vi "Example.vi"() -> ()   [LabVIEW 2020]
doc: "Modbus RTU for Invertek drives. Paul Nathan 21-JUN-2022."
uses:
  ctls/Drive address.ctl
  ctls/Modbus error cluster.ctl
  ctls/Exception codes.ctl
panel:
  out "No errors":bool
  out "Modbus error cluster":T1={"Checksum ok"=FALSE, "Modbus exception code"=1, "Response from correct drive"=FALSE, "Comms error"={"status"=FALSE, "code"=0, "source"=""}} {"Modbus exception code" items=["None"=0, "Invalid function request"=1, "Invalid Modbus register address"=2, "Invalid / unauthorised data value"=3, "Device failure"=4, "Request accepted, wait"=5, "Drive busy"=6, "Request rejected"=7, "Memory parity error"=8, "Gateway path unavailable"=10, "Device failed to respond"=11]}
  out "Motor power (kW)":dbl
  in  "Drive address":T3=1 items=["0", "1", "2", "3", "4", "5", "6", "7", "8", "9", "10", "11", "12", "13", "14", "15", "16", "17", "18", "19", "20", "21", "22", "23", "24", "25", "26", "27", "28", "29", "30", "31", "32", "33", "34", "35", "36", "37", "38", "39", "40", "41", "42", "43", "44", "45", "46", "47", "48", "49", "50", "51", "52", "53", "54", "55", "56", "57", "58", "59", "60", "61", "62", "63"]
  in  "COM port":refnum<visa-resource-name>
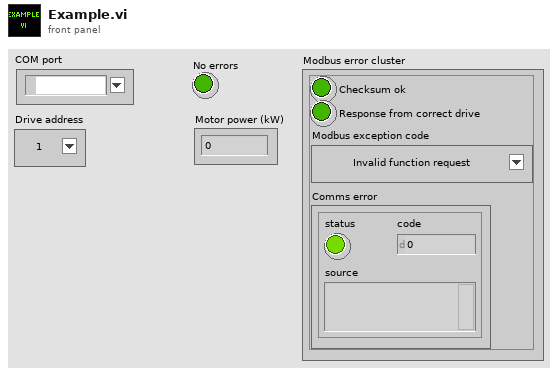
[diagram p1: front panel]
types:
  T1 = typedef "Modbus error cluster.ctl" = cluster{"Checksum ok":bool, "Modbus exception code":T2, "Response from correct drive":bool, "Comms error":errorcluster}
  T2 = typedef "Exception codes.ctl" = u8
  T3 = typedef "Drive address.ctl" = u8
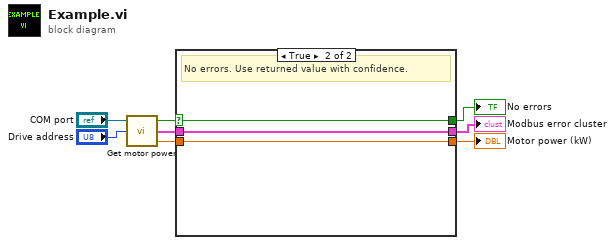
[diagram p0: block diagram]
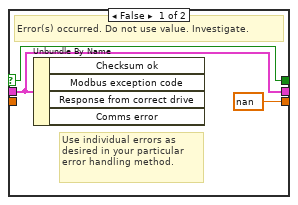
[diagram p2: hidden frame]
diagram:
  n1 = call "Get motor power.vi"("Drive address"="Drive address", "COM port"="COM port") -> ("Motor power (kW)"=w5:dbl, "Modbus error cluster"=w3:T1, "No errors"=w6:bool)  [unwired: 1 in]
  n2 = case shown="True" w6 {
    selector: w6 -> [w9 w12]
    tunnel: w5 -> [_ w14]
    tunnel: [nan ("Motor power (kW)") w14] -> w4
    tunnel: w3 -> [w10 w13]
    tunnel: [w10 w13] -> w2
    tunnel: [w9 w12] -> w1
    frame False {
      # "Use individual errors as desired in your particular error handling method."
      # "Error(s) occurred. Do not use value. Investigate."
      n3 = Unbundle By Name(w10) -> ()  [unwired: 4 out]
    }
    frame True {
      # "No errors. Use returned value with confidence."
    }
  }
  "Motor power (kW)" <- w4
  "Modbus error cluster" <- w2
  "No errors" <- w1
